vi "test.vi"() -> ()   [LabVIEW 2015]
panel:
  in  "Physical Channel":refnum<k21>="Dev1/Ai0"
  out "Waveform Chart":waveform(dbl)(graph)
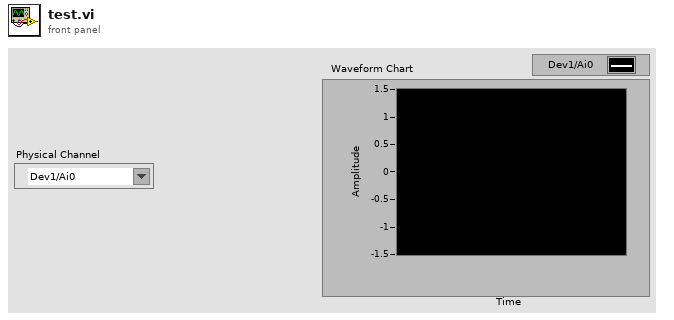
[diagram p1: front panel]
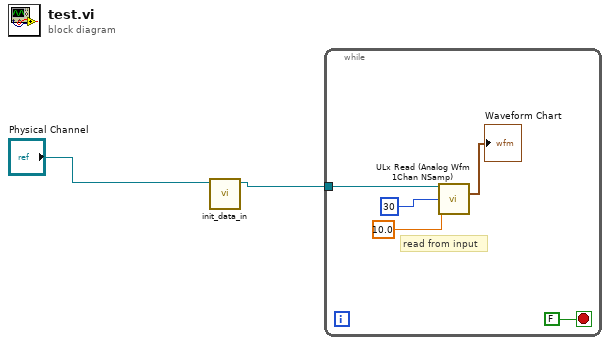
[diagram p0: block diagram]
diagram:
  n1 = call "init_data_in.vi"("output channel"="Physical Channel") -> ("task out"=w1:refnum<k24>)  [unwired: 9 in, 1 out]
  n2 = while {
    tunnel: w1 -> [w4]
    stop <- FALSE stop-if-true
    # "read from input"
    n3 = call <vilib>:"ULx Read (Analog Wfm 1Chan NSamp).vi"("task in"=w4, "number of samples per channel"=30 ("samples per channel"), "timeout"=10.0) -> ("data"=→"Waveform Chart":waveform(dbl))  [unwired: 10 in, 2 out]
  }
